vi "Plot Spectrum.vi"(8 "error in (no error)":errorcluster, 11 "Micron Optics Recorder in":refnum<class "Micron Optics Recorder.lvclass">) -> (0 "error out":errorcluster, 3 "Micron Optics Recorder out":refnum<class "Micron Optics Recorder.lvclass">)   [LabVIEW 2016, in "Micron Optics Recorder.lvclass"]
uses:
  Micron Optics Recorder.lvclass
  NHMFL_Core/Libraries/Instruments/Micron Optics/Micron Optics Driver/Micron Optics Driver.lvclass
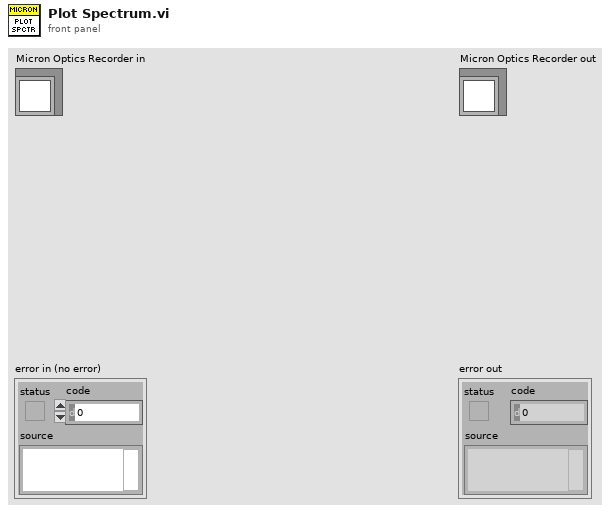
[diagram p1: front panel]
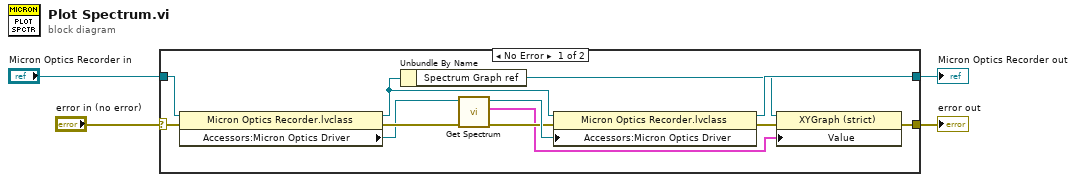
[diagram p0: block diagram]
diagram:
  n1 = case shown="No Error" "error in (no error)" {
    selector: "error in (no error)" -> [w16 w18]
    tunnel: [w7 w18] -> w3
    tunnel: [w11 w17] -> w1
    tunnel: "Micron Optics Recorder in" -> [w14 w17]
    frame No Error {
      n2 = property class="Micron Optics Recorder.lvclass"(reference=w14, error in=w16) -> (reference out=w8:refnum<class "Micron Optics Recorder.lvclass">, error out=w15:errorcluster, "Accessors:Micron Optics Driver"=w13:refnum<class "Micron Optics Driver.lvclass">)
      n3 = Unbundle By Name(w8) -> ("Spectrum Graph ref"=w6:refnum<vi>)
      n4 = call-dynamic "Get Spectrum.vi"("error in (no error)"=w15, "Micron Optics Driver in"=w13) -> ("error out"=w9:errorcluster, "Spectrum Graph"=w5:cluster{dbl[], "Spectrum, db":dbl[]}[], "Micron Optics Driver out"=w10:refnum<class "Micron Optics Driver.lvclass">)  [unwired: 7 in]
      n5 = property class="Micron Optics Recorder.lvclass"(reference=w8, error in=w9, "Accessors:Micron Optics Driver"=w10) -> (reference out=w11:refnum<class "Micron Optics Recorder.lvclass">, error out=w12:errorcluster)
      n6 = property class="XYGraph (strict)"(reference=w6, error in=w12, "Value"=w5) -> (error out=w7:errorcluster)  [unwired: 1 out]
    }
    frame Error {
    }
  }
  "error out" <- w3
  "Micron Optics Recorder out" <- w1
